vi "State_machine_server.vi"() -> ()   [LabVIEW 2010]
uses:
  <vilib>/Utility/tcp.llb/TCP Listen.vi
panel:
  out "ror 2":bool
  out "boyle 2":bool
  out "Ventil 2":bool=TRUE
  out "ror 1":bool
  out "boyle 1":bool
  out "Ventil 1":bool=TRUE
  in  "Port":u16
  out "Nød modus":bool
  out "Normalmodus":bool
  in  "STOPP programmet":bool
  in  "Pause prosess":bool
  in  "Fyller og Tømmer":bool
  in  "Hastighet [L/s]":dbl(knob) scale=0.0..100.0
  out "Nød-styring":bool
  in  "Server styring":bool
  out "Remote IP-adresse":string
  out "Prosess stoppet":bool
  out "Tomt":bool
  out "Fullt":bool
  out "Tømmer":bool
  out "Fyller":bool
  out "Vertsnavn":string
  out "IP-adresse, string. Dot-notasjon":string
  out "Tank":dbl(slide) scale=0.0..1000.0
  out "Tilstand":T1(ring)
  # "Liter med vann"
  # "Fyller"
  # "Hastighet [L/s]"
  # "Tømmer"
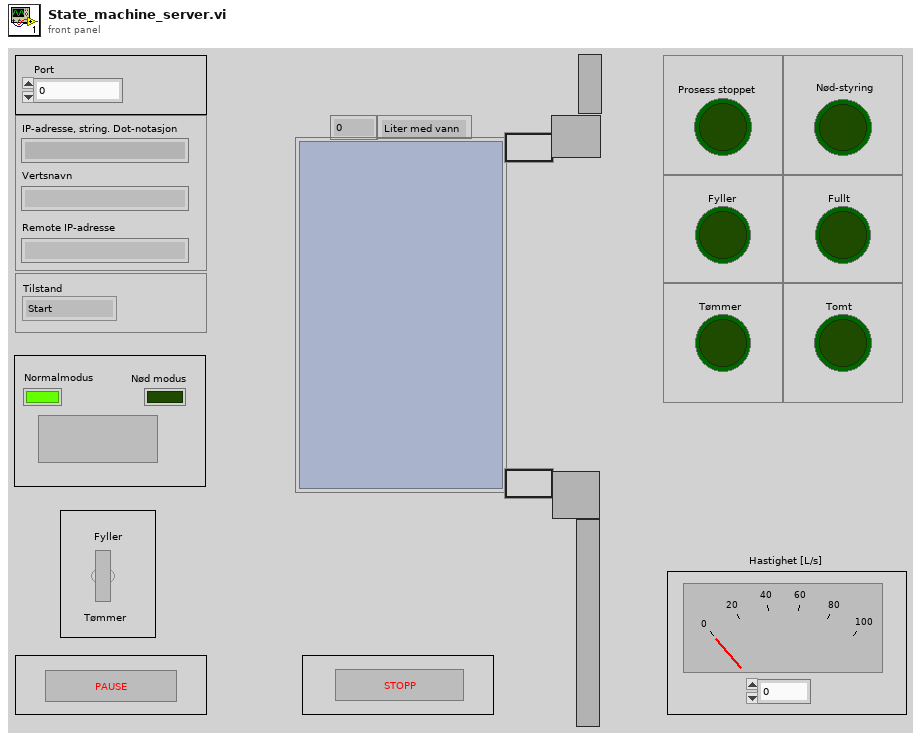
[diagram p1: front panel]
types:
  T1 = enum16{"Start", "Tomt", "Fyller", "Tømmer", "Fullt", "Stopp"}
  T2 = enum16{"Standard", "Buffered", "CRLF", "Immediate"}
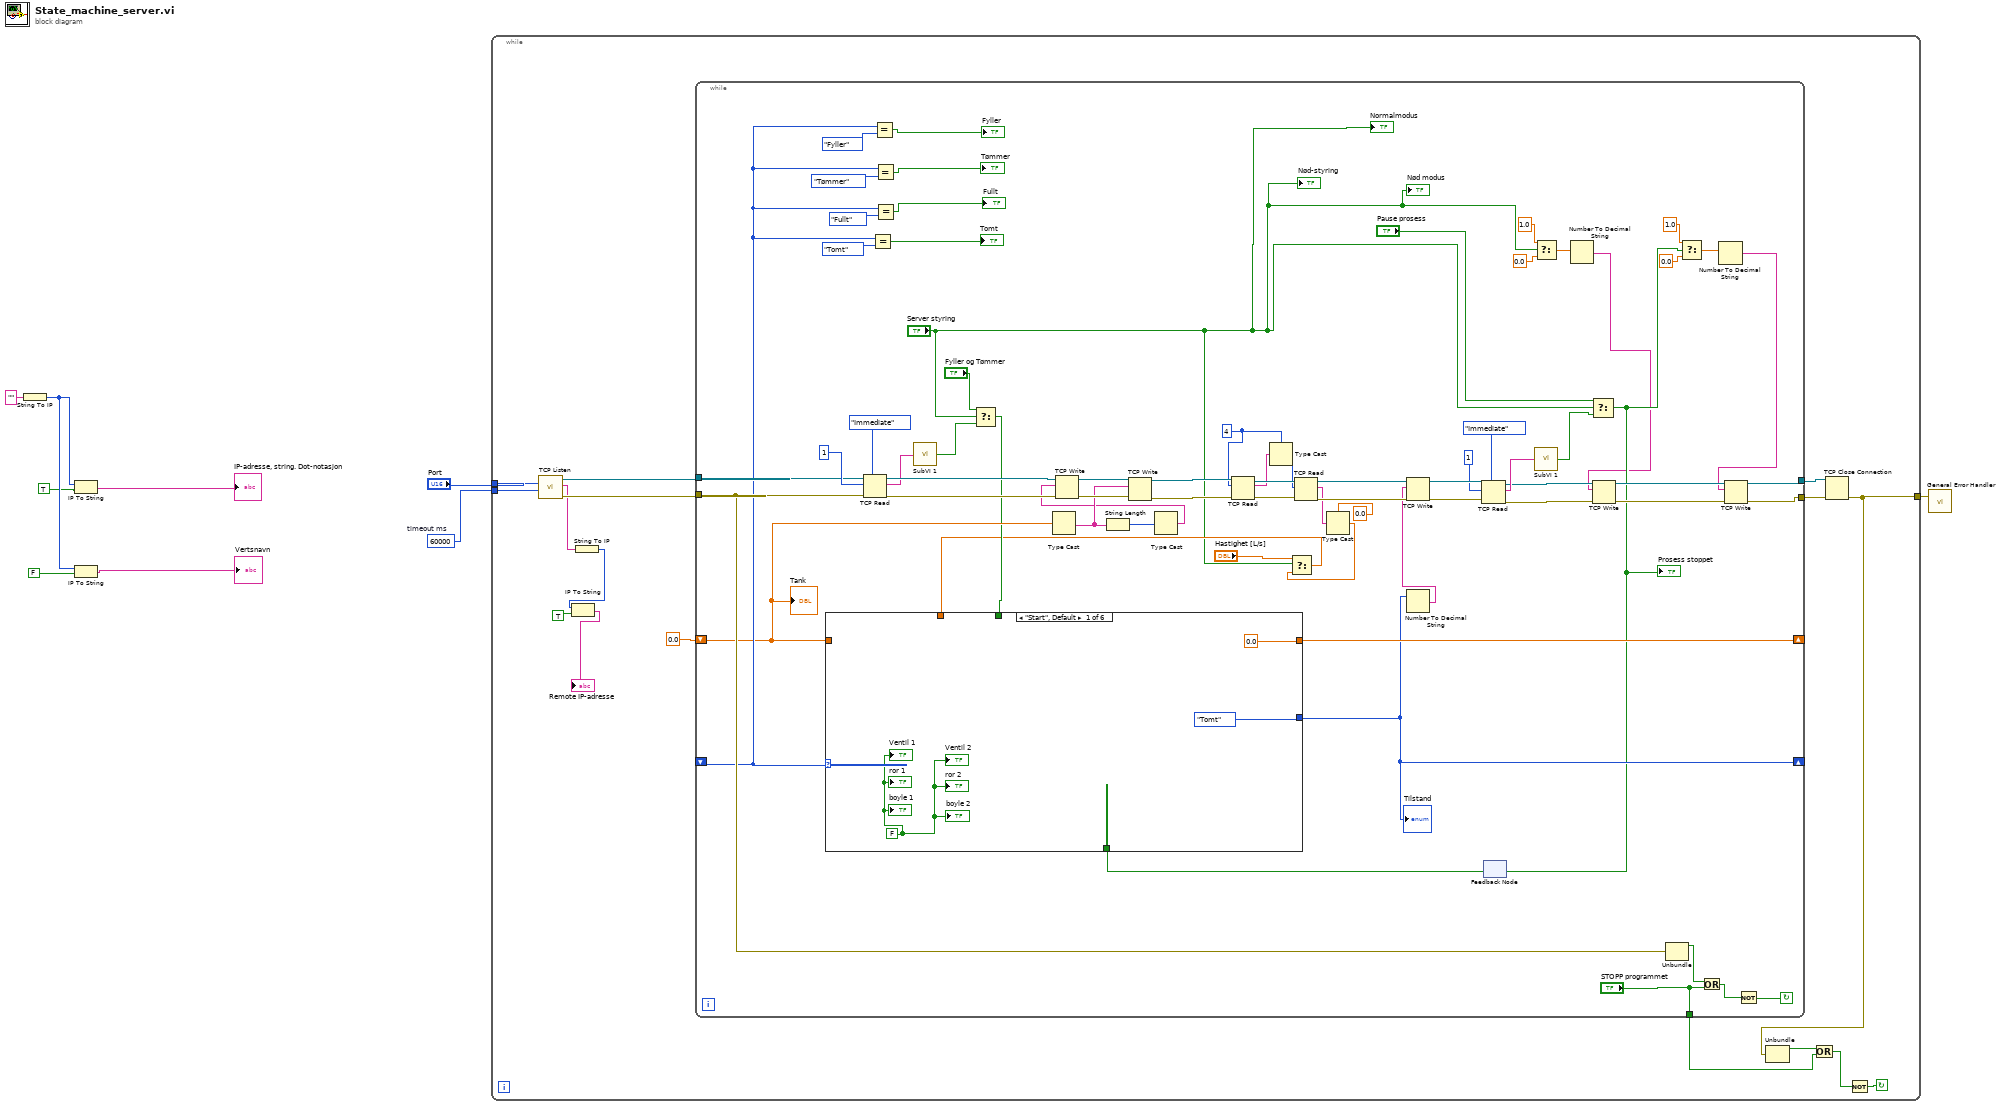
[diagram p0: block diagram]
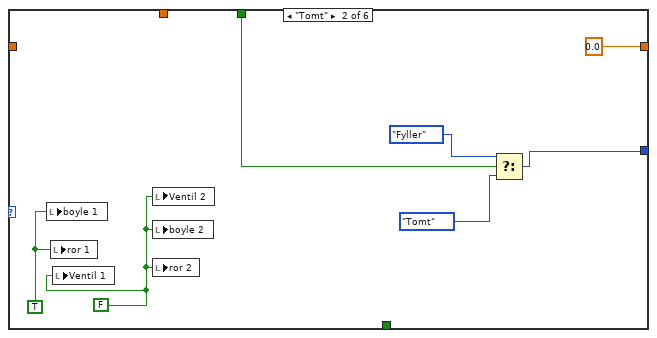
[diagram p2: hidden frame]
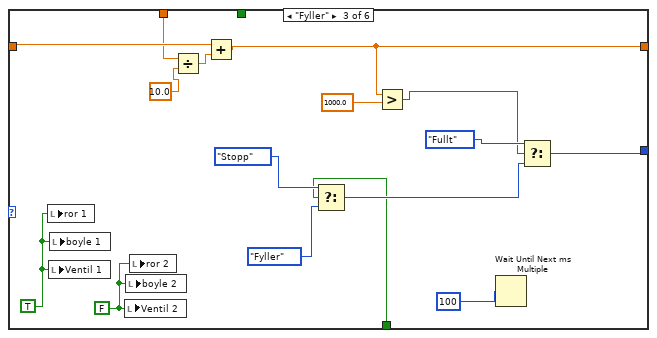
[diagram p3: hidden frame]
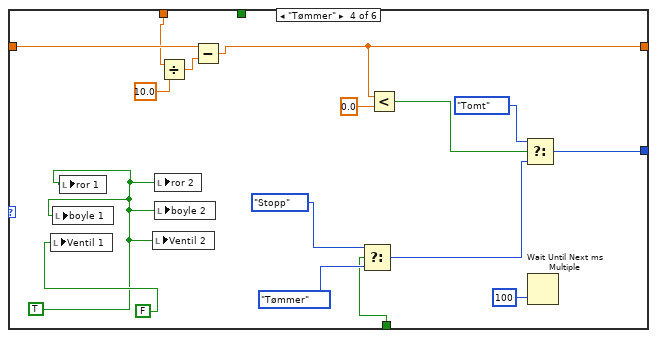
[diagram p4: hidden frame]
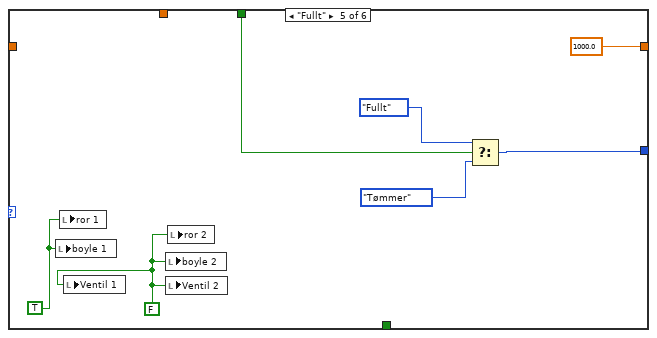
[diagram p5: hidden frame]
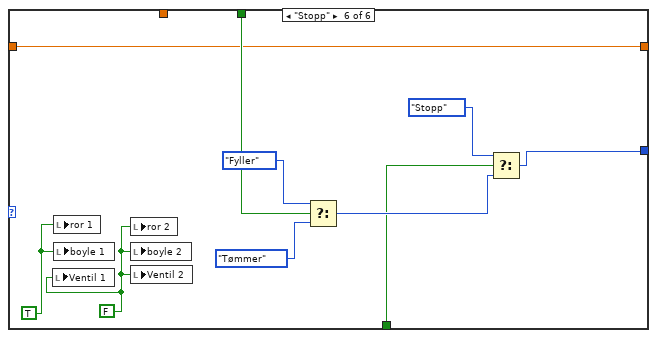
[diagram p6: hidden frame]
diagram:
  w8 = 60000  # timeout ms
  n1 = String To IP(1:"" ("name")) -> (0:w5:u32)
  n2 = IP To String(1:TRUE, 2:w5) -> (0:→"IP-adresse, string. Dot-notasjon":string)
  n3 = IP To String(1:FALSE, 2:w5) -> (0:→"Vertsnavn":string)
  n4 = while {
    tunnel: "Port" -> [w14]
    tunnel: [w11] -> w9
    tunnel: w8 -> [w19]
    stop <- w17 continue-if-true
    n5 = call "TCP Listen"("timeout ms (wait forever: -1)"=w19, "port"=w14) -> ("error out"=w24:errorcluster, "remote address"=w13:string, "connection ID"=w23:refnum<k5>)  [unwired: 6 in, 1 out]
    n6 = String To IP(1:w13) -> (0:w18:u32)
    n7 = IP To String(1:TRUE, 2:w18) -> (0:→"Remote IP-adresse":string)
    n8 = while {
      shift-right: [w95] -> _
      shift-left: 0.0 -> [w48]
      shift-right: [w87] -> _
      shift-left: _ -> [w49]
      tunnel: w24 -> [w50]
      tunnel: w23 -> [w82]
      tunnel: [w40] -> w22
      tunnel: ["STOPP programmet"] -> w16
      tunnel: [w39] -> w15
      stop <- w61 continue-if-true
      w35 = 4 ("bytes to read")
      n9 = TCP Read(connection ID=w82, bytes to read=1, error in (no error)=w50, 7:T2."Immediate" ("mode (standard)")) -> (connection ID out=w94:refnum<k5>, data out=w47:string, error out=w93:errorcluster)  [unwired: 1 in]
      n10 = Equal?(x=w49, y=T1."Tomt") -> (x = y?=→"Tomt":bool)
      n11 = Equal?(x=w49, y=T1."Fyller") -> (x = y?=→"Fyller":bool)
      n12 = Equal?(x=w49, y=T1."Tømmer") -> (x = y?=→"Tømmer":bool)
      n13 = Equal?(x=w49, y=T1."Fullt") -> (x = y?=→"Fullt":bool)
      n14 = call "SubVI 1.vi"("Input string"=w47) -> ("Output boolean"=w45:bool)
      n15 = Select(t="Fyller og Tømmer", s="Server styring", f=w45) -> (s? t:f=w46:bool)
      n16 = Type Cast(x=w48) -> (*(type *) &x=w89:string)  [unwired: 1 in]
      n17 = String Length(string=w89) -> (length=w88:i32)
      n18 = Type Cast(x=w88) -> (*(type *) &x=w43:string)  [unwired: 1 in]
      n19 = TCP Write(connection ID=w94, data in=w43, error in (no error)=w93) -> (connection ID out=w91:refnum<k5>, error out=w90:errorcluster)  [unwired: 1 in, 1 out]
      n20 = TCP Write(connection ID=w91, data in=w89, error in (no error)=w90) -> (connection ID out=w73:refnum<k5>, error out=w78:errorcluster)  [unwired: 1 in, 1 out]
      n21 = TCP Read(connection ID=w73, bytes to read=w35, error in (no error)=w78) -> (connection ID out=w74:refnum<k5>, data out=w72:string, error out=w77:errorcluster)  [unwired: 2 in]
      n22 = Type Cast(type=w35, x=w72) -> (*(type *) &x=w71:i32)
      n23 = TCP Read(connection ID=w74, bytes to read=w71, error in (no error)=w77) -> (connection ID out=w75:refnum<k5>, data out=w32:string, error out=w76:errorcluster)  [unwired: 2 in]
      n24 = Type Cast(type=0.0, x=w32) -> (*(type *) &x=w33:dbl)
      n25 = Select(t="Hastighet [L/s]", s="Server styring", f=w33) -> (s? t:f=w34:dbl)
      n26 = feedback #1() -> (w81:bool)  [unwired: 1 in]
      n27 = case shown="\"Start\", Default" w49 {
        tunnel: [0.0 0.0 w112 w124 1000.0 w145] -> w95
        tunnel: [T1."Tomt" w105 w121 w136 w143 w154] -> w87
        tunnel: w48 -> [_ _ w111 w125 _ w145]
        tunnel: w46 -> [_ w101 _ _ w140 w149]
        tunnel: w81 -> [_ _ w113 w129 _ w148]
        tunnel: w34 -> [_ _ w108 w122 _ _]
        frame "Start", Default {
          w96 = FALSE
          "Ventil 1" <- w96
          "ror 1" <- w96
          "boyle 1" <- w96
          "Ventil 2" <- w96
          "boyle 2" <- w96
          "ror 2" <- w96
        }
        frame "Tomt" {
          w100 = TRUE
          w99 = FALSE
          n28 = local write "boyle 1"(w100) -> ()
          n29 = local write "ror 1"(w100) -> ()
          n30 = local write "Ventil 1"(w99) -> ()
          n31 = local write "Ventil 2"(w99) -> ()
          n32 = local write "boyle 2"(w99) -> ()
          n33 = local write "ror 2"(w99) -> ()
          n34 = Select(t=T1."Fyller", s=w101, f=T1."Tomt") -> (s? t:f=w105:T1)
        }
        frame "Fyller" {
          w107 = FALSE
          w106 = TRUE
          n35 = local write "ror 1"(w106) -> ()
          n36 = local write "Ventil 1"(w106) -> ()
          n37 = local write "boyle 1"(w106) -> ()
          n38 = local write "Ventil 2"(w107) -> ()
          n39 = local write "boyle 2"(w107) -> ()
          n40 = local write "ror 2"(w107) -> ()
          n41 = Divide(x=w108, y=10.0) -> (x/y=w110:dbl)
          n42 = Add(x=w111, y=w110) -> (x+y=w112:dbl)
          n43 = Select(t=T1."Stopp", s=w113, f=T1."Fyller") -> (s? t:f=w120:T1)
          n44 = Greater?(x=w112, y=1000.0) -> (0:w115:bool)
          n45 = Wait Until Next ms Multiple(millisecond multiple=u32 100) -> ()  [unwired: 1 out]
          n46 = Select(t=T1."Fullt", s=w115, f=w120) -> (s? t:f=w121:T1)
        }
        frame "Tømmer" {
          w126 = TRUE
          n47 = local write "Ventil 1"(FALSE) -> ()
          n48 = local write "boyle 1"(w126) -> ()
          n49 = local write "ror 1"(w126) -> ()
          n50 = local write "Ventil 2"(w126) -> ()
          n51 = local write "ror 2"(w126) -> ()
          n52 = local write "boyle 2"(w126) -> ()
          n53 = Divide(x=w122, y=10.0) -> (x/y=w128:dbl)
          n54 = Subtract(x=w125, y=w128) -> (x-y=w124:dbl)
          n55 = Select(t=T1."Stopp", s=w129, f=T1."Tømmer") -> (s? t:f=w135:T1)
          n56 = Less?(x=w124, y=0.0) -> (x < y?=w133:bool)
          n57 = Select(t=T1."Tomt", s=w133, f=w135) -> (s? t:f=w136:T1)
          n58 = Wait Until Next ms Multiple(millisecond multiple=u32 100) -> ()  [unwired: 1 out]
        }
        frame "Fullt" {
          w139 = FALSE
          w138 = TRUE
          n59 = local write "boyle 1"(w138) -> ()
          n60 = local write "ror 1"(w138) -> ()
          n61 = local write "Ventil 1"(w139) -> ()
          n62 = local write "boyle 2"(w139) -> ()
          n63 = local write "Ventil 2"(w139) -> ()
          n64 = local write "ror 2"(w139) -> ()
          n65 = Select(t=T1."Fullt", s=w140, f=T1."Tømmer") -> (s? t:f=w143:T1)
        }
        frame "Stopp" {
          w146 = TRUE
          w147 = FALSE
          n66 = local write "Ventil 1"(w147) -> ()
          n67 = local write "ror 1"(w146) -> ()
          n68 = local write "boyle 1"(w146) -> ()
          n69 = local write "ror 2"(w147) -> ()
          n70 = local write "boyle 2"(w147) -> ()
          n71 = local write "Ventil 2"(w147) -> ()
          n72 = Select(t=T1."Fyller", s=w149, f=T1."Tømmer") -> (s? t:f=w153:T1)
          n73 = Select(t=T1."Stopp", s=w148, f=w153) -> (s? t:f=w154:T1)
        }
      }
      "Tilstand" <- w87
      n74 = Number To Decimal String(number=w87) -> (decimal integer string=w28:string)  [unwired: 1 in]
      n75 = TCP Write(connection ID=w75, data in=w28, error in (no error)=w76) -> (connection ID out=w86:refnum<k5>, error out=w85:errorcluster)  [unwired: 1 in, 1 out]
      n76 = TCP Read(connection ID=w86, bytes to read=1, error in (no error)=w85, 7:T2."Immediate" ("mode (standard)")) -> (connection ID out=w58:refnum<k5>, data out=w79:string, error out=w57:errorcluster)  [unwired: 1 in]
      n77 = Select(t=1.0, s="Server styring", f=0.0) -> (s? t:f=w38:dbl)
      n78 = call "SubVI 1.vi"("Input string"=w79) -> ("Output boolean"=w37:bool)
      n79 = Number To Decimal String(number=w38) -> (decimal integer string=w27:string)  [unwired: 1 in]
      n80 = Select(t="Pause prosess", s="Server styring", f=w37) -> (s? t:f=w42:bool)
      "Prosess stoppet" <- w42
      n81 = feedback-in #1(w42) -> ()
      n82 = TCP Write(connection ID=w58, data in=w27, error in (no error)=w57) -> (connection ID out=w54:refnum<k5>, error out=w53:errorcluster)  [unwired: 1 in, 1 out]
      n83 = Unbundle "Unbundle"(w50) -> ("status"=w44:bool)  [unwired: 2 out]
      n84 = Select(t=1.0, s=w42, f=0.0) -> (s? t:f=w41:dbl)
      n85 = Or(x=w44, y="STOPP programmet") -> (x .or. y?=w60:bool)
      n86 = Number To Decimal String(number=w41) -> (decimal integer string=w26:string)  [unwired: 1 in]
      n87 = TCP Write(connection ID=w54, data in=w26, error in (no error)=w53) -> (connection ID out=w40:refnum<k5>, error out=w39:errorcluster)  [unwired: 1 in, 1 out]
      n88 = Not(x=w60) -> (.not. x?=w61:bool)
      "Tank" <- w48
      "Nød-styring" <- "Server styring"
      "Nød modus" <- "Server styring"
      "Normalmodus" <- "Server styring"
    }
    n89 = TCP Close Connection(connection ID=w22, error in (no error)=w15) -> (error out=w11:errorcluster)  [unwired: 1 in, 1 out]
    n90 = Unbundle(w11) -> ("status"=w10:bool)  [unwired: 2 out]
    n91 = Or(x=w10, y=w16) -> (x .or. y?=w12:bool)
    n92 = Not(x=w12) -> (.not. x?=w17:bool)
  }
  n93 = call <vilib>:"General Error Handler.vi"("error in (no error)"=w9) -> ()  [unwired: 10 in, 5 out]
